vi "ProducerConsumerData (Multiple Queues).vi"() -> ()   [LabVIEW 2019]
doc: "Use this template to build a producer/consumer design pattern. Use this template when you need to execute a process, such as data analysis, when a data source, such as a triggered acquisition, produces data at an uneven rate and you need to execute the process when the data becomes available."
panel:
  out "data (can be any type) 2":string
  out "data (can be any type)":string
  in  "stop":bool
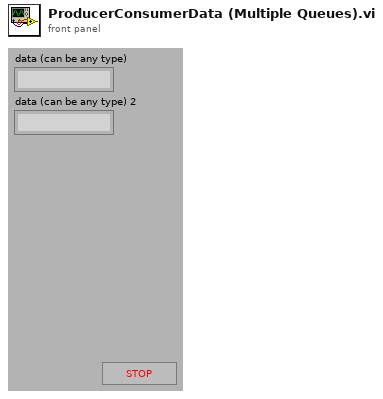
[diagram p1: front panel]
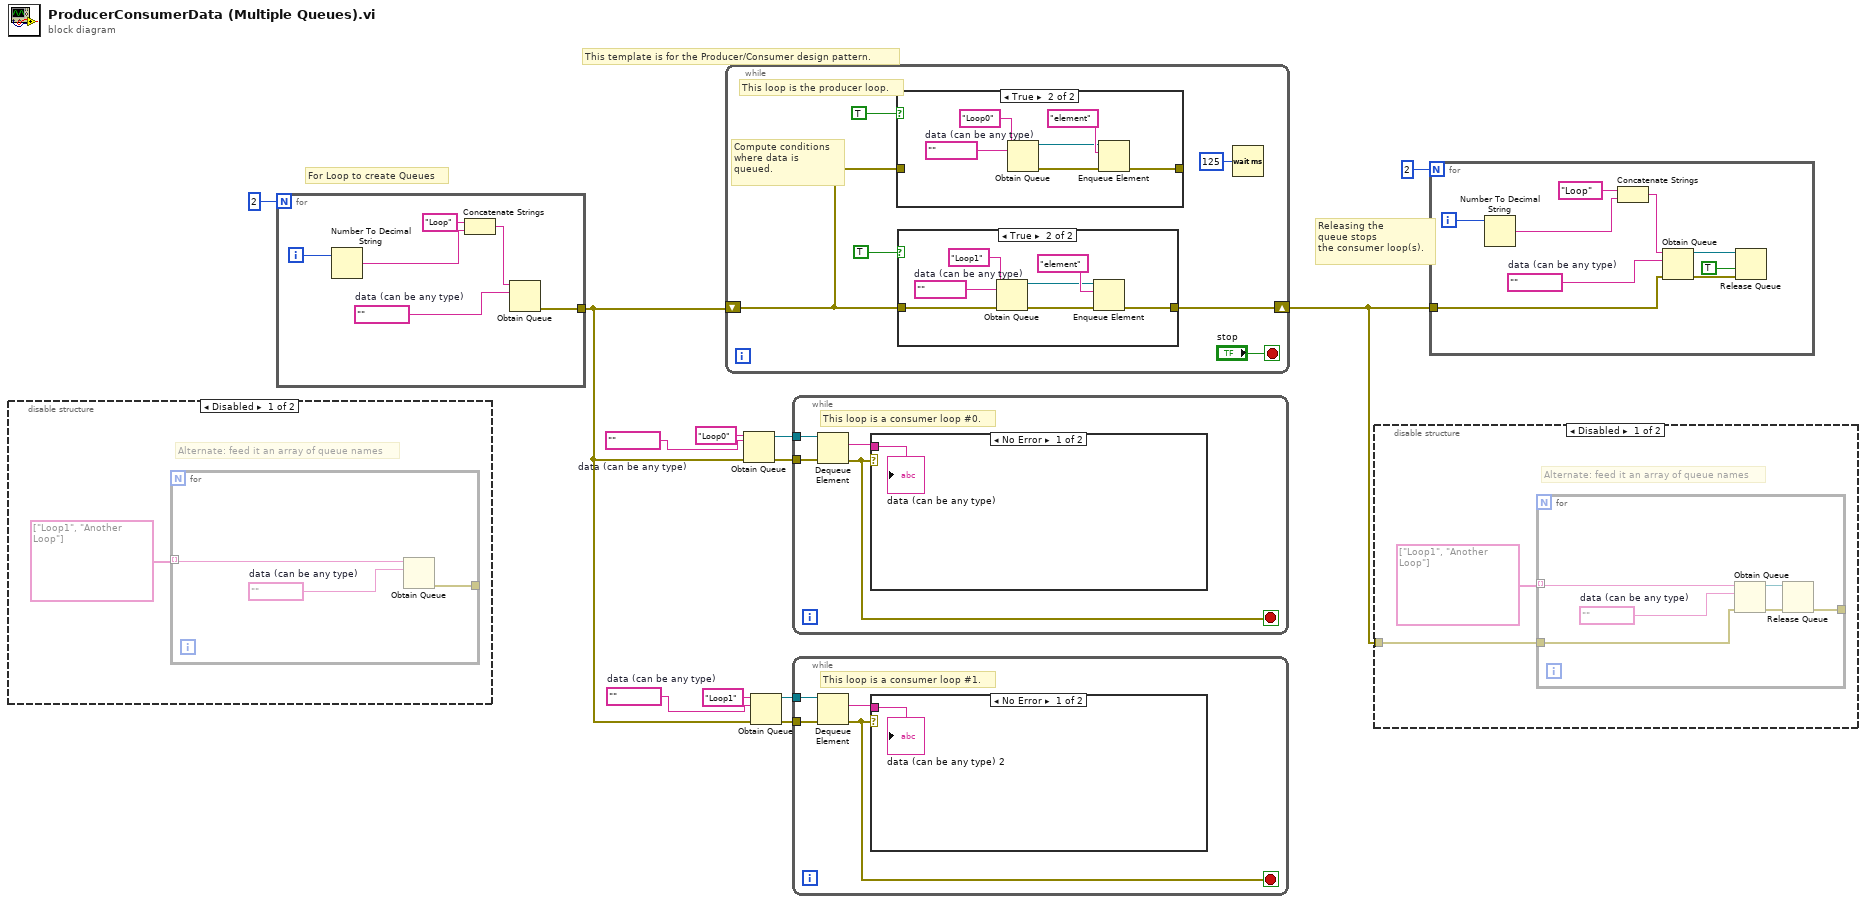
[diagram p0: block diagram]
diagram:
  w7 = ""  # data (can be any type)
  w8 = ""  # data (can be any type)
  # "For Loop to create Queues"
  # "Releasing the\nqueue stops\nthe consumer loop(s)."
  # "This template is for the Producer/Consumer design pattern."
  n1 = disable-structure shown="Disabled" {
    frame Disabled {
      # "Alternate: feed it an array of queue names"
      n2 = for {
        tunnel: [w16] -> _
        tunnel: string[] ["Loop1", "Another Loop"] -> [w14] mode=indexing
        w15 = ""  # data (can be any type)
        n3 = Obtain Queue(name (unnamed)=w14, element data type=w15) -> (error out=w16:errorcluster)  [unwired: 3 in, 2 out]
      }
    }
    frame Enabled {
    }
  }
  n4 = for {
    N: 2 -> [_]
    tunnel: [w22] -> w2
    i -> [w17]
    w21 = ""  # data (can be any type)
    n5 = Number To Decimal String(number=w17) -> (decimal integer string=w19:string)  [unwired: 1 in]
    n6 = Concatenate Strings("Loop" ("string"), w19) -> (w18:string)
    n7 = Obtain Queue(name (unnamed)=w18, element data type=w21) -> (error out=w22:errorcluster)  [unwired: 3 in, 2 out]
  }
  n8 = while {
    shift-right: [w23] -> w1
    shift-left: w2 -> [w24]
    stop <- "stop" stop-if-true
    # "Compute conditions\nwhere data is\nqueued."
    # "This loop is the producer loop."
    n9 = case shown="True" TRUE {
      tunnel: [w29 w35] -> _
      tunnel: w24 -> [w29 _]
      frame False {
      }
      frame True {
        w32 = ""  # data (can be any type)
        n10 = Obtain Queue(name (unnamed)="Loop0", element data type=w32) -> (queue out=w30:refnum<queue>, error out=w31:errorcluster)  [unwired: 3 in, 1 out]
        n11 = Enqueue Element(queue=w30, element="element", error in (no error)=w31) -> (error out=w35:errorcluster)  [unwired: 1 in, 2 out]
      }
    }
    n12 = case shown="True" TRUE ("Case Constant\n(See Context Help)") {
      tunnel: w24 -> [w36 w40]
      tunnel: [w36 w43] -> w23
      frame False {
      }
      frame True {
        w38 = ""  # data (can be any type)
        n13 = Obtain Queue(name (unnamed)="Loop1", element data type=w38, error in (no error)=w40) -> (queue out=w41:refnum<queue>, error out=w39:errorcluster)  [unwired: 2 in, 1 out]
        n14 = Enqueue Element(queue=w41, element="element", error in (no error)=w39) -> (error out=w43:errorcluster)  [unwired: 1 in, 2 out]
      }
    }
    n15 = Wait (ms)(milliseconds to wait=u32 125) -> ()  [unwired: 1 out]
  }
  n16 = Obtain Queue(name (unnamed)="Loop0", element data type=w8, error in (no error)=w2) -> (queue out=w10:refnum<queue>, error out=w9:errorcluster)  [unwired: 2 in, 1 out]
  n17 = Obtain Queue(name (unnamed)="Loop1", element data type=w7, error in (no error)=w2) -> (queue out=w5:refnum<queue>, error out=w4:errorcluster)  [unwired: 2 in, 1 out]
  n18 = while {
    tunnel: w10 -> [w47]
    tunnel: w9 -> [w45]
    stop <- w46 stop-if-true
    # "This loop is a consumer loop #0."
    n19 = Dequeue Element(queue=w47, error in (no error)=w45) -> (element=w44:string, error out=w46:errorcluster)  [unwired: 1 in, 2 out]
    n20 = case shown="No Error" w46 {
      tunnel: w44 -> [w48 _]
      frame No Error {
        "data (can be any type)" <- w48
      }
      frame Error {
      }
    }
  }
  n21 = while {
    tunnel: w5 -> [w51]
    tunnel: w4 -> [w50]
    stop <- w52 stop-if-true
    # "This loop is a consumer loop #1."
    n22 = Dequeue Element(queue=w51, error in (no error)=w50) -> (element=w49:string, error out=w52:errorcluster)  [unwired: 1 in, 2 out]
    n23 = case shown="No Error" w52 {
      tunnel: w49 -> [w53 _]
      frame No Error {
        "data (can be any type) 2" <- w53
      }
      frame Error {
      }
    }
  }
  n24 = disable-structure shown="Disabled" {
    disable-tunnel: w1 -> [w54 _]
    frame Disabled {
      # "Alternate: feed it an array of queue names"
      n25 = for {
        tunnel: [w58] -> _
        tunnel: string[] ["Loop1", "Another Loop"] -> [w59] mode=indexing
        tunnel: w54 -> [w56]
        w60 = ""  # data (can be any type)
        n26 = Obtain Queue(name (unnamed)=w59, element data type=w60, error in (no error)=w56) -> (queue out=w57:refnum<queue>, error out=w61:errorcluster)  [unwired: 2 in, 1 out]
        n27 = Release Queue(queue=w57, error in (no error)=w61) -> (error out=w58:errorcluster)  [unwired: 1 in, 2 out]
      }
    }
    frame Enabled {
    }
  }
  n28 = for {
    N: 2 -> [_]
    tunnel: w1 -> [w66]
    i -> [w63]
    w70 = ""  # data (can be any type)
    n29 = Number To Decimal String(number=w63) -> (decimal integer string=w68:string)  [unwired: 1 in]
    n30 = Concatenate Strings("Loop" ("string"), w68) -> (w67:string)
    n31 = Obtain Queue(name (unnamed)=w67, element data type=w70, error in (no error)=w66) -> (queue out=w64:refnum<queue>, error out=w65:errorcluster)  [unwired: 2 in, 1 out]
    n32 = Release Queue(queue=w64, force destroy? (F)=TRUE, error in (no error)=w65) -> ()  [unwired: 3 out]
  }
